vi "Read movement.vi"(8 "error in (no error)":errorcluster, 11 "BabyHuman in":refnum<class "BabyHuman.lvclass">) -> (0 "error out":errorcluster, 2 "movement":string, 3 "BabyHuman out":refnum<class "BabyHuman.lvclass">)   [LabVIEW 2017, in "BabyHuman.lvclass"]
uses:
  BabyHuman.lvclass
  BabyHuman.lvclass/BabyHuman.ctl
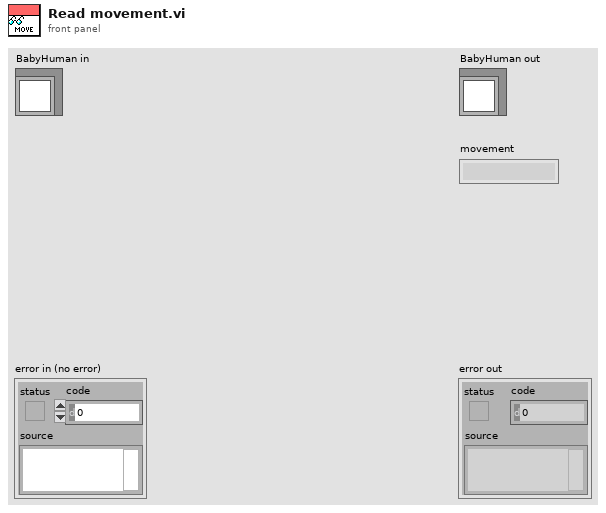
[diagram p1: front panel]
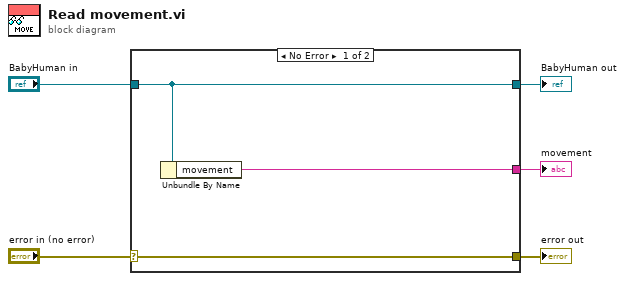
[diagram p0: block diagram]
diagram:
  n1 = case shown="No Error" "error in (no error)" {
    selector: "error in (no error)" -> [w8 w9]
    tunnel: [w8 w9] -> w4
    tunnel: [w7 w10] -> w2
    tunnel: "BabyHuman in" -> [w7 w10]
    tunnel: [w6 _] -> w1
    frame No Error {
      n2 = Unbundle By Name(w7) -> ("movement"=w6:string)
    }
    frame Error {
    }
  }
  "error out" <- w4
  "BabyHuman out" <- w2
  "movement" <- w1
